vi "Update Position.vi"(8 "error in (no error)":errorcluster, 9 "Direction":T1, 10 "Action":T2, 11 "Sentinel in":refnum<class "Sentinel.lvclass">) -> (0 "error out":errorcluster, 2 "Sentinel in 2":refnum<class "Sentinel.lvclass">, 3 "Sentinel out":refnum<class "Sentinel.lvclass">)   [LabVIEW 2020, in "Sentinel.lvclass"]
uses:
  Sentinel.lvclass
  Type Defs/Action Enum.ctl
  Type Defs/Direction Enum.ctl
  Sentinel.lvclass/Sentinel.ctl
  Type Defs/SB Type Defs.lvlib
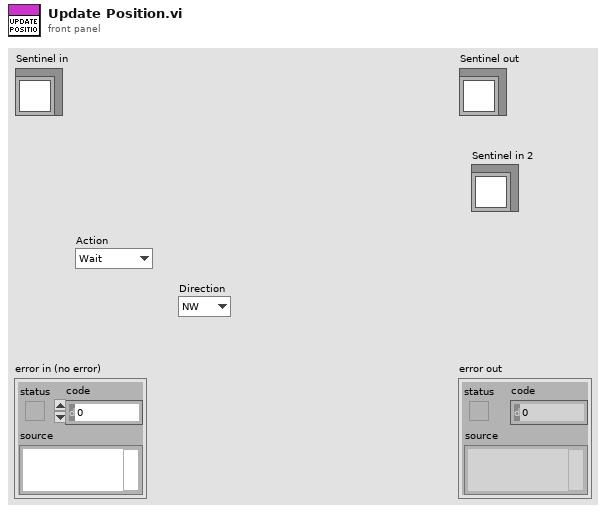
[diagram p1: front panel]
types:
  T1 = typedef "SB Type Defs.lvlib/Direction Enum.ctl" = enum16{"NW", "N", "NE", "E", "SE", "S", "SW", "W"}
  T2 = typedef "SB Type Defs.lvlib/Action Enum.ctl" = enum16{"Wait", "Move", "Attack", "Replicate"}
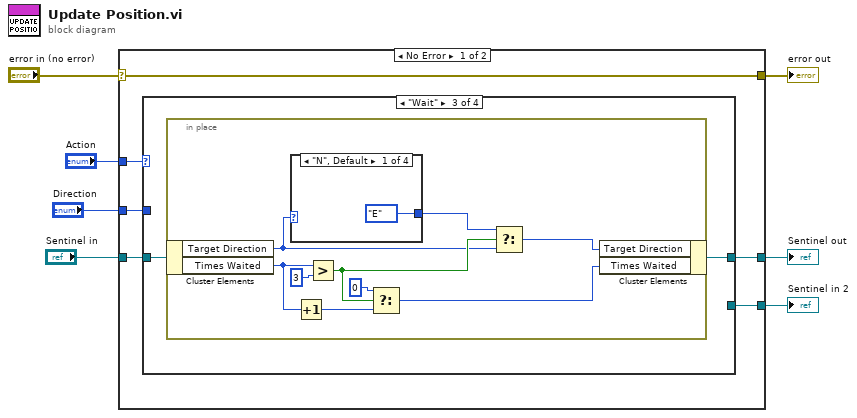
[diagram p0: block diagram]
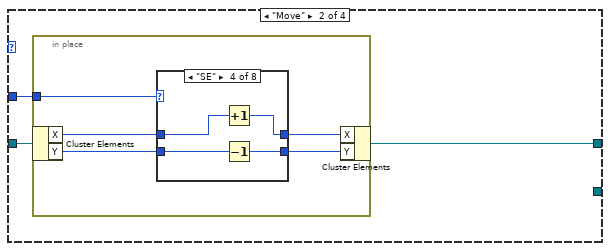
[diagram p3: hidden frame]
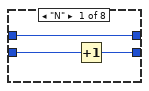
[diagram p4: hidden frame]
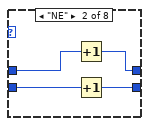
[diagram p5: hidden frame]
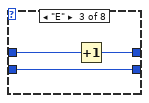
[diagram p6: hidden frame]
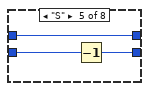
[diagram p7: hidden frame]
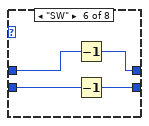
[diagram p8: hidden frame]
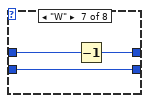
[diagram p9: hidden frame]
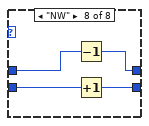
[diagram p10: hidden frame]
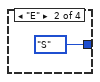
[diagram p11: hidden frame]
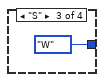
[diagram p12: hidden frame]
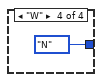
[diagram p13: hidden frame]
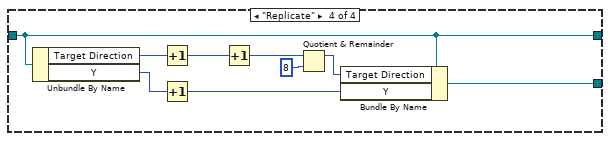
[diagram p14: hidden frame]
diagram:
  n1 = case shown="No Error" "error in (no error)" {
    selector: "error in (no error)" -> [w13 w76]
    tunnel: [w13 w76] -> w6
    tunnel: [w10 w75] -> w4
    tunnel: "Sentinel in" -> [w11 w75]
    tunnel: "Action" -> [w12 _]
    tunnel: [w9 _] -> w2
    tunnel: "Direction" -> [w8 _]
    frame No Error {
      n2 = case shown="\"Wait\"" w12 {
        tunnel: w11 -> [w14 w16 w52 w73]
        tunnel: [w14 w15 w51 w73] -> w10
        tunnel: [_ _ _ w74] -> w9
        tunnel: w8 -> [_ w17 _ _]
        frame Default {
        }
        frame "Move" {
          n3 = in-place {
            in-place-border: w17 -> [w22]
            n4 = in-place-cluster #1(w16) -> ("X"=w21:i16, "Y"=w20:i16)
            n5 = case shown="\"SE\"" w22 {
              tunnel: w21 -> [w25 w29 w32 w36 w39 w43 w46 w50]
              tunnel: w20 -> [w24 w28 w31 w35 w38 w42 w45 w49]
              tunnel: [w25 w27 w30 w33 w39 w41 w44 w47] -> w19
              tunnel: [w23 w26 w31 w34 w37 w40 w45 w48] -> w18
              frame "N" {
                n6 = Increment(x=w24) -> (x+1=w23:i16)
              }
              frame "NE" {
                n7 = Increment(x=w29) -> (x+1=w27:i16)
                n8 = Increment(x=w28) -> (x+1=w26:i16)
              }
              frame "E" {
                n9 = Increment(x=w32) -> (x+1=w30:i16)
              }
              frame "SE" {
                n10 = Increment(x=w36) -> (x+1=w33:i16)
                n11 = Decrement(x=w35) -> (x-1=w34:i16)
              }
              frame "S" {
                n12 = Decrement(x=w38) -> (x-1=w37:i16)
              }
              frame "SW" {
                n13 = Decrement(x=w43) -> (x-1=w41:i16)
                n14 = Decrement(x=w42) -> (x-1=w40:i16)
              }
              frame "W" {
                n15 = Decrement(x=w46) -> (x-1=w44:i16)
              }
              frame "NW" {
                n16 = Decrement(x=w50) -> (x-1=w47:i16)
                n17 = Increment(x=w49) -> (x+1=w48:i16)
              }
            }
            n18 = in-place-cluster #1("X"=w19, "Y"=w18) -> (w15:refnum<class "Sentinel.lvclass">)
          }
        }
        frame "Wait" {
          n19 = in-place {
            n20 = in-place-cluster #2(w52) -> ("Target Direction"=w54:T1, "Times Waited"=w60:i8)
            n21 = case shown="\"N\", Default" w54 {
              tunnel: [Direction_Enum."E" ("Direction") Direction_Enum."S" ("Direction") Direction_Enum."W" ("Direction") Direction_Enum."N" ("Direction")] -> w53
              frame "N", Default {
              }
              frame "E" {
              }
              frame "S" {
              }
              frame "W" {
              }
            }
            n22 = Increment(x=w60) -> (x+1=w59:i8)
            n23 = Greater?(x=w60, y=i8 3) -> (0:w56:bool)
            n24 = Select(t=i8 0, s=w56, f=w59) -> (s? t:f=w57:i8)
            n25 = Select(t=w53, s=w56, f=w54) -> (s? t:f=w55:T1)
            n26 = in-place-cluster #2("Target Direction"=w55, "Times Waited"=w57) -> (w51:refnum<class "Sentinel.lvclass">)
          }
        }
        frame "Replicate" {
          n27 = Unbundle By Name(w73) -> ("Target Direction"=w67:T1, "Y"=w72:i16)
          n28 = Increment(x=w67) -> (x+1=w66:T1)
          n29 = Increment(x=w72) -> (x+1=w71:i16)
          n30 = Increment(x=w66) -> (x+1=w70:T1)
          n31 = Quotient & Remainder(x=w70, y=8) -> (x-y*floor(x/y)=w68:i32)  [unwired: 1 out]
          n32 = Bundle By Name(cluster=w73, "Target Direction"=w68, "Y"=w71) -> (w74:refnum<class "Sentinel.lvclass">)
        }
      }
    }
    frame Error {
    }
  }
  "error out" <- w6
  "Sentinel out" <- w4
  "Sentinel in 2" <- w2
